vi "Get Pressure.vi"() -> (2 "Voltage":dbl)   [LabVIEW 2014]
uses:
  Robot Global Data.vi
panel:
  out "Pressure":dbl
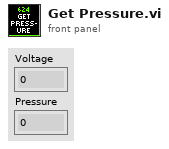
[diagram p1: front panel]
types:
  T1 = typedef "Dashboard Control Data.ctl" = cluster{"Cam Exposure":dbl, "Go to angle":dbl, "PID gains":cluster{"proportional gain (Kc)":dbl, "integral time (Ti, min)":dbl, "derivative time (Td, min)":dbl}, "output range":cluster{"output high":dbl, "output low":dbl}, "Pressure m \nValue":dbl, "Pressure b \nValue":dbl}
  T2 = typedef "WPI_AnalogChannelDevRef.ctl" = cluster{"DevStatus":errorcluster, "Controller":T3, "Analog Channel":T4}
  T3 = typedef "FPGA_TypedefAnalogModule.ctl" = enum16{"Controller 1"}
  T4 = typedef "FPGA_AIChannel.ctl" = enum8{"AI 0", "AI 1", "AI 2", "AI 3", "AI MXP 0", "AI MXP 1", "AI MXP 2", "AI MXP 3", "Invalid"}
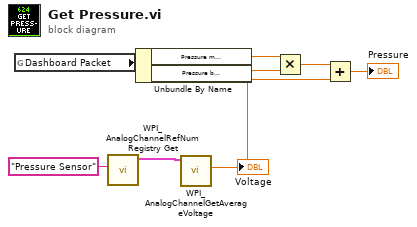
[diagram p0: block diagram]
diagram:
  n1 = global read "Robot Global Data.vi" "Dashboard Packet"() -> (w6:T1)
  n2 = call <vilib>:"WPI_AnalogChannelRefNum Registry Get.vi"("refnum name"="Pressure Sensor") -> ("AIDeviceRef"=w8:T2)  [unwired: 9 in, 1 out]
  n3 = Unbundle By Name(w6) -> ("Pressure m \nValue"=w5:dbl, "Pressure b \nValue"=w3:dbl)
  n4 = call <vilib>:"WPI_AnalogChannelGetAverageVoltage.vi"("AIDeviceRef"=w8) -> ("Voltage"=w4:dbl)  [unwired: 8 in, 2 out]
  "Voltage" <- w4
  n5 = Multiply(x=w5, y=w4) -> (x*y=w2:dbl)
  n6 = Add(x=w2, y=w3) -> (x+y=→"Pressure":dbl)
